vi "Process.vi"(8 "error in":errorcluster, 11 "Framework-Template":refnum<class "Instrument.Framework-Template.lvclass">) -> (0 "error out":errorcluster, 3 "Framework-Template out":refnum<class "Instrument.Framework-Template.lvclass">)   [LabVIEW 2019, in "Instrument.Framework-Template.lvclass"]
doc: "---------------------------------------------------------------\nJKI State Machine Objects™\nhttp://jki.net/state-machine-objects/\nCopyright (C) 2005-2015, JKI <info@jki.net>\nALL RIGHTS RESERVED"
uses:
  Instrument.Framework-Template.lvclass
  <vilib>/JKI/JKI SMO/SMO/SMO.lvclass
  Framework/Instrument/Instrument.lvclass
  C:/Users/patrick/Documents/GitHub/Instrument-Framework/lvsrc/Framework/Instrument Types/SCPI/Instrument.SCPI.lvclass
  C:/Users/patrick/Documents/GitHub/Instrument-Framework/lvsrc/Framework/Instrument/Instrument.lvclass
  C:/Program Files (x86)/National Instruments/LabVIEW 2019/vi.lib/JKI/JKI SMO/SMO/SMO.lvclass
  <userlib>/LevyLab/RemoteControl/RemoteControl/Typedefs/Message--Cluster.ctl
  <userlib>/LevyLab/RemoteControl/RemoteControl/RemoteControl.lvclass
  Typedefs/PrivateEvents--Framework-Template.MessageToProcess.ctl
  Framework/Instrument Types/SCPI/Instrument.SCPI.lvclass
  subsystems/HAL/HAL.lvclass
panel:
  out "Status":string
  out "State History":string
  # "Instrument.Framework-Template"
  # "Framework-Template"
  # "For instructions on how to use the JKI State Machine Objects, examples and video tutorials, visit:\nhttp://jki.net/state-machine-objects/\n\nJKI State Machine Objects™\nhttp://jki.net/state-machine-objects/\nCopyright (C) 2005-2015, JKI <info@jki.net>\nALL RIGHTS RESERVED"
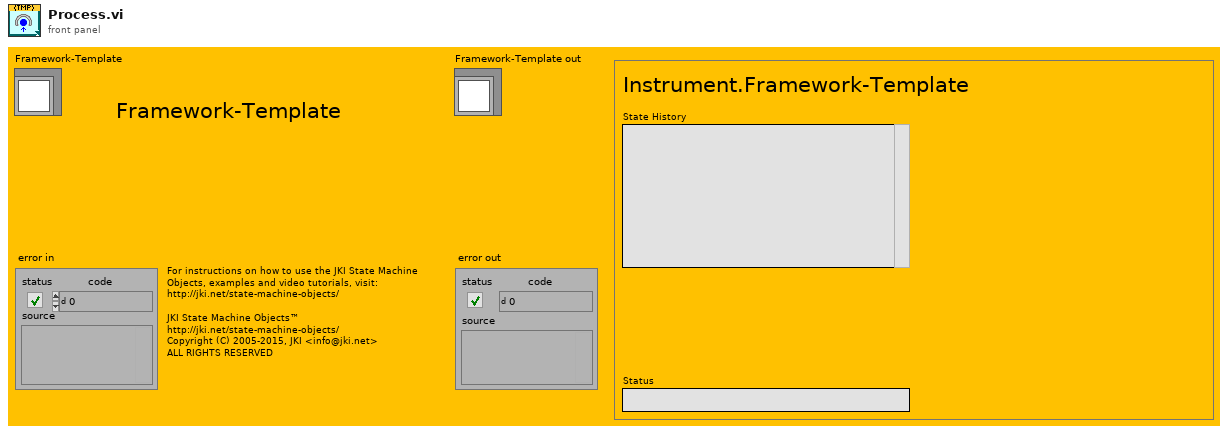
[diagram p1: front panel]
types:
  T1 = enum32{"invalid app kind", "Development System", "Run Time System", "Student Edition", "Embedded LabVIEW", "Evaluation", "Custom"}
  T2 = enum32{"Invalid", "Standard", "Closed", "Hidden", "Minimized", "Maximized"}
  T3 = typedef "RemoteControl.lvclass/Message--Cluster.ctl" = cluster{"Command":string, "Data":variant, "ID":string}
  T4 = typedef "Instrument.Framework-Template.lvclass/PrivateEvents--Framework-Template.MessageToProcess.ctl" = cluster{"Message":T3}
  T5 = cluster{"Core":cluster{"Current VI Reference":refnum<vi>, "Close Panel on Exit?":bool, "Last Error":cluster{"error":errorcluster, "previous state":string, "remaining states":string}, "Shutdown?":bool}, "SelfRef":refnum<class "Instrument.Framework-Template.lvclass">, "HAL":refnum<class "HAL.lvclass">, "Running Step":i32, "sequence":string[], "MessageToProcess":T4}
  T6 = cluster{"Current VI Reference":refnum<vi>, "Close Panel on Exit?":bool, "Last Error":cluster{"error":errorcluster, "previous state":string, "remaining states":string}, "Shutdown?":bool}
  T7 = typedef "SMO.lvclass/Protected Events.ctl" = cluster{"StopProcesses":refnum<user-event>, "AbortProcesses":refnum<user-event>, "Config Changed":refnum<user-event>, "Dependency":refnum<user-event>}
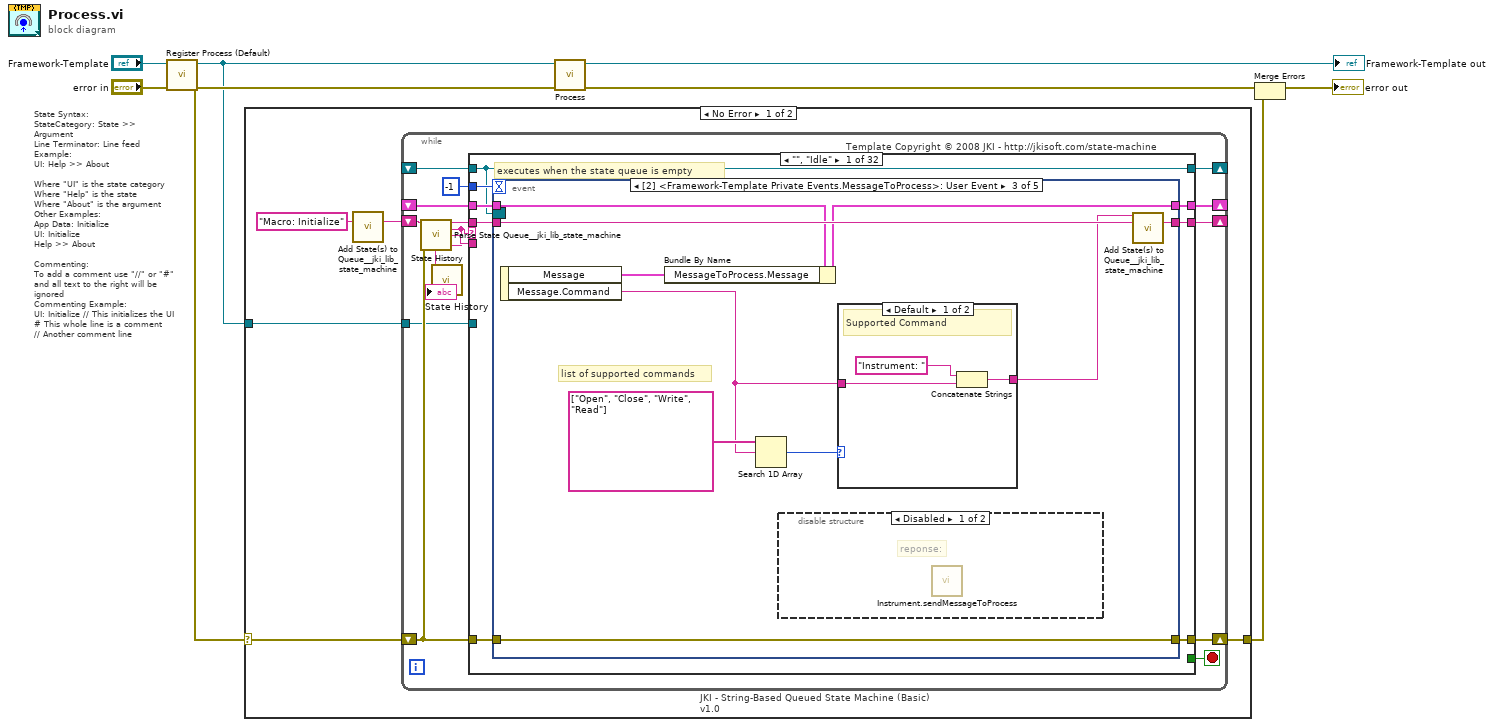
[diagram p0: block diagram]
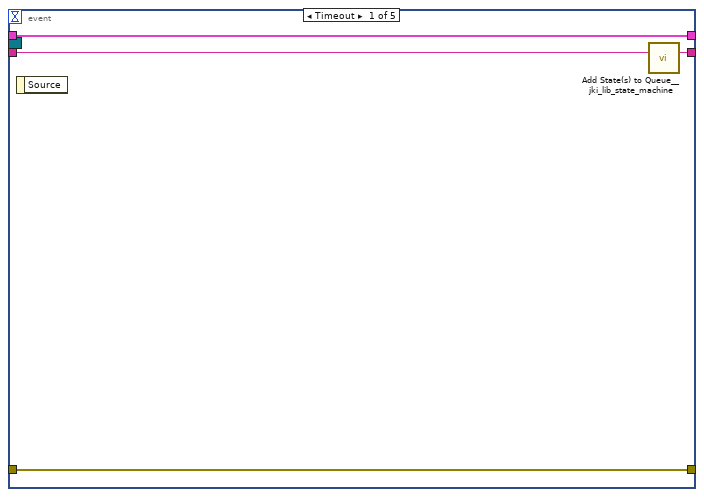
[diagram p2: hidden frame]
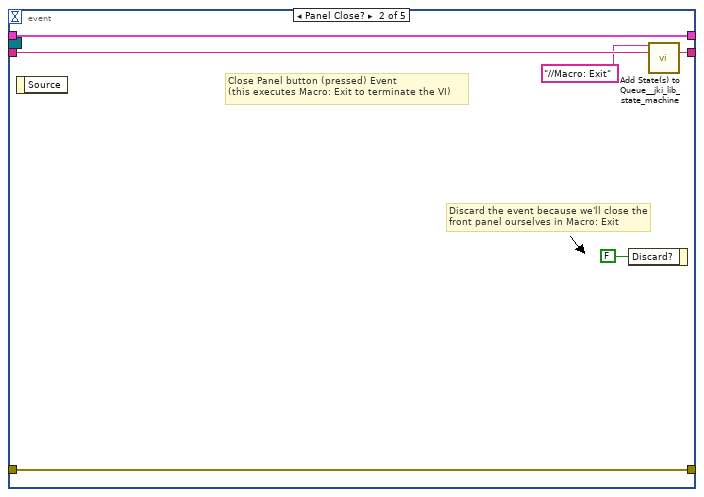
[diagram p3: hidden frame]
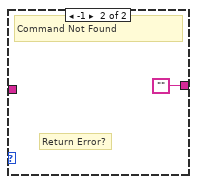
[diagram p5: hidden frame]
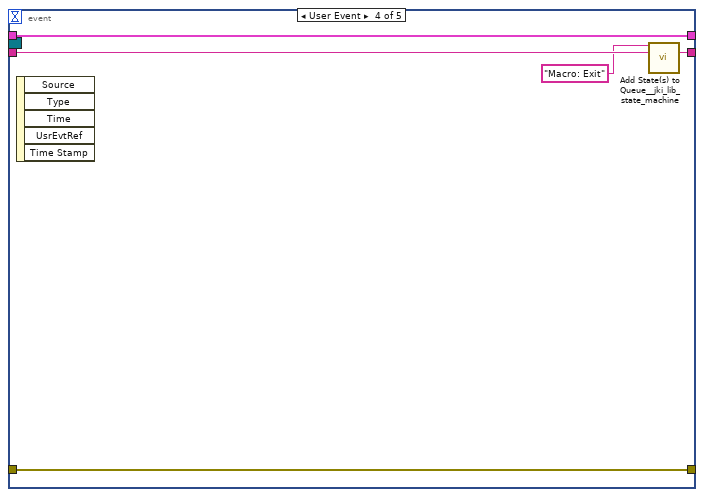
[diagram p6: hidden frame]
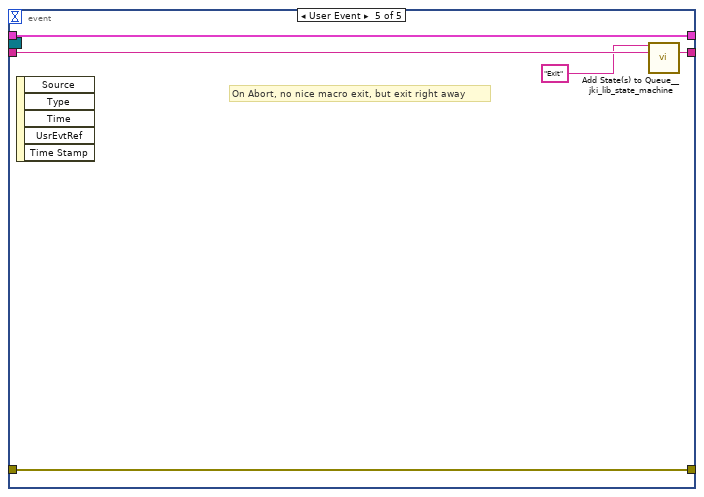
[diagram p7: hidden frame]
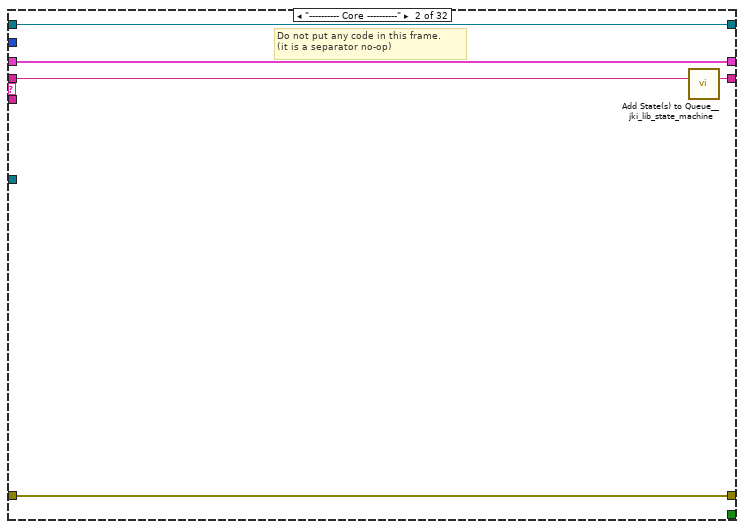
[diagram p8: hidden frame]
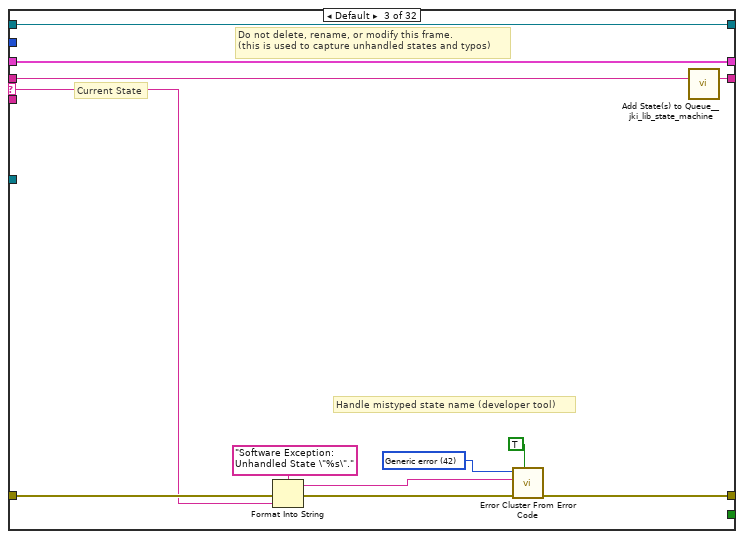
[diagram p9: hidden frame]
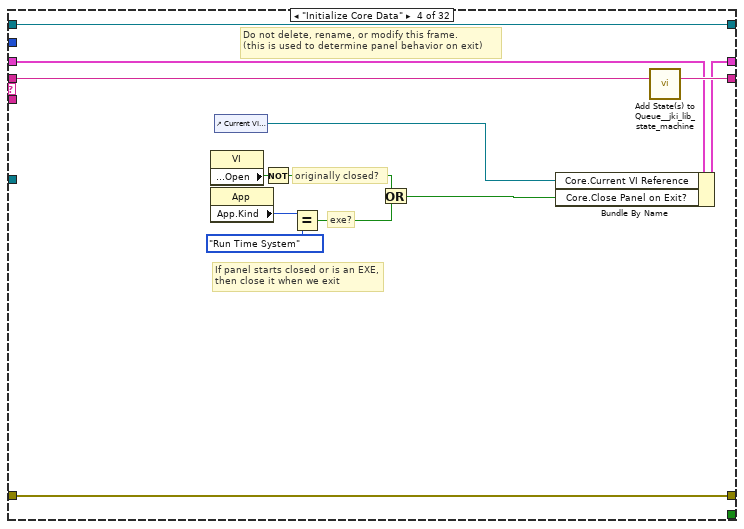
[diagram p10: hidden frame]
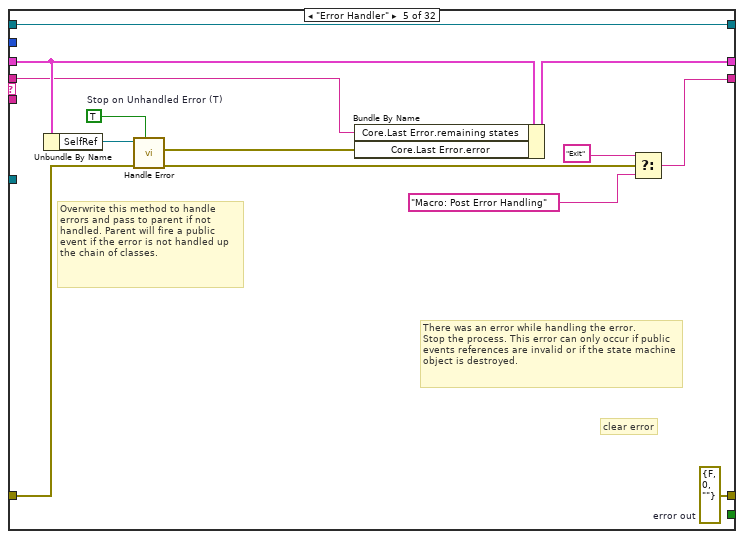
[diagram p11: hidden frame]
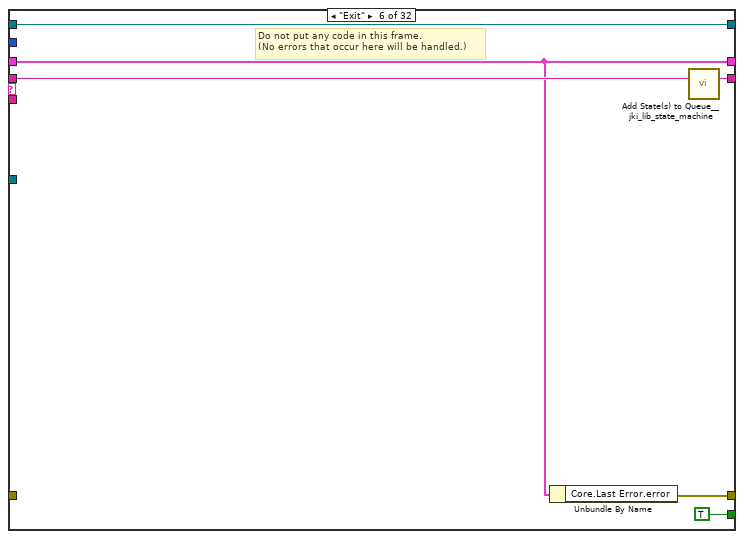
[diagram p12: hidden frame]
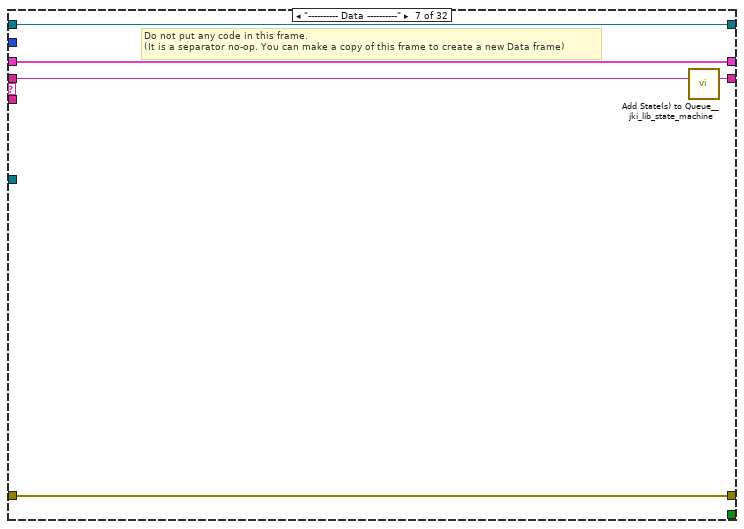
[diagram p13: hidden frame]
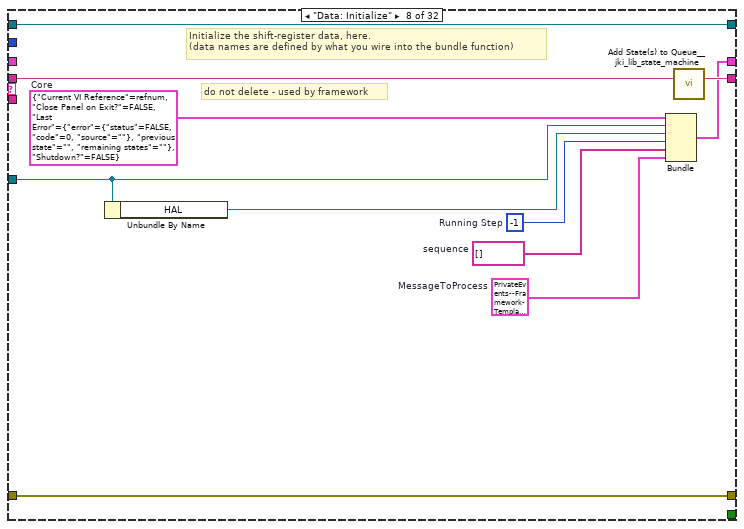
[diagram p14: hidden frame]
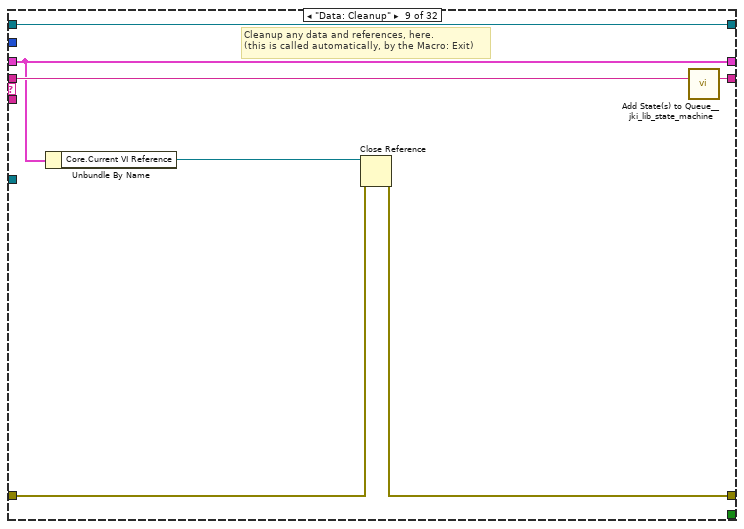
[diagram p15: hidden frame]
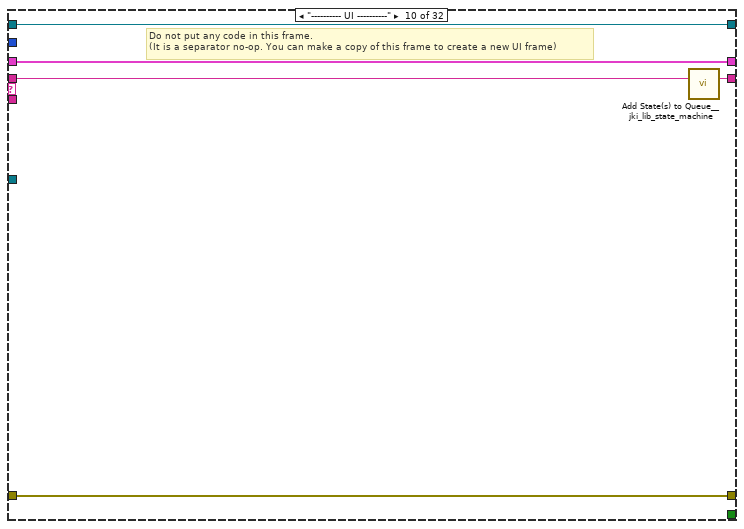
[diagram p16: hidden frame]
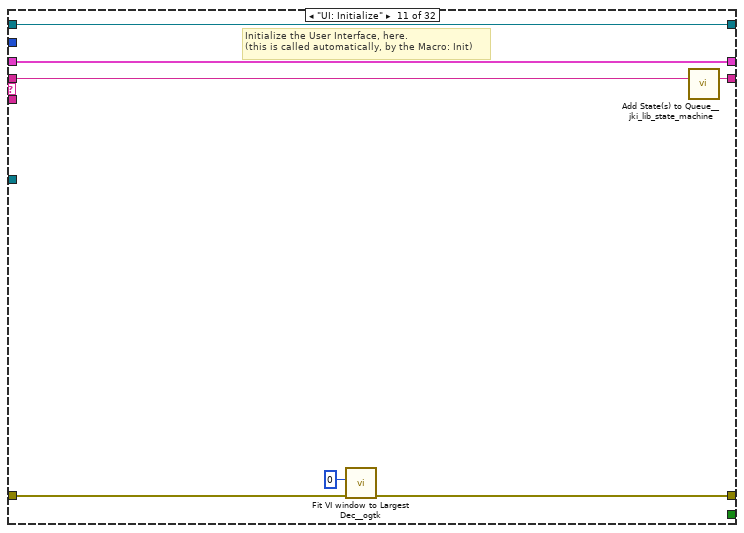
[diagram p17: hidden frame]
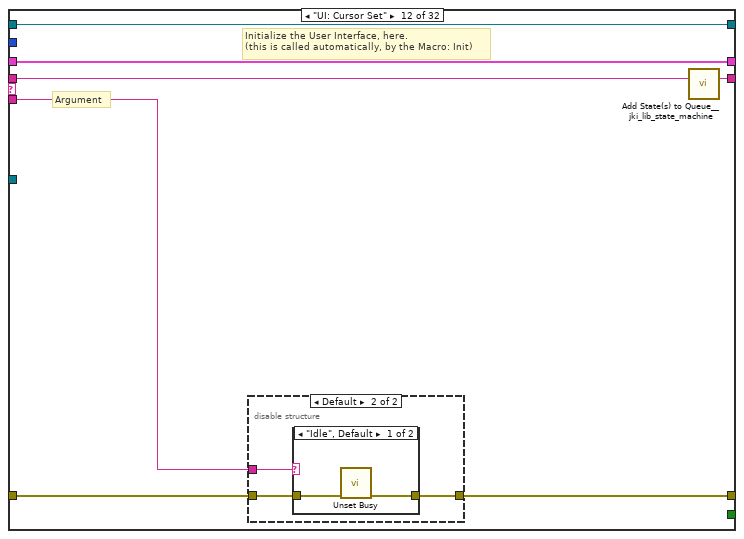
[diagram p18: hidden frame]
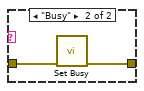
[diagram p20: hidden frame]
diagram:
  # "State Syntax:\nStateCategory: State >> Argument\nLine Terminator: Line feed\nExample:\nUI: Help >> About\n\nWhere \"UI\" is the state category\nWhere \"Help\" is the state\nWhere \"About\" is the argument\nOther Examples:\nApp Data: Initialize\nUI: Initialize\nHelp >> About\n\nCommenting:\nTo add a comment use \"//\" or \"#\" and all text to the right will be ignored\nCommenting Example:\nUI: Initialize // This initializes the UI\n# This whole line is a comment\n// Another comment line"
  n1 = call <vilib>:"Register Process (Default).vi"("error in (no error)"="error in", "SMO"="Framework-Template") -> ("error out"=w5:errorcluster, "SelfRef"=w4:refnum<class "Instrument.Framework-Template.lvclass">)  [unwired: 8 in]
  n2 = case shown="No Error" w5 {
    selector: w5 -> [w10 w422]
    tunnel: w4 -> [w11 _]
    tunnel: [w9 w422] -> w1
    frame No Error {
      n3 = call <vilib>:"Add State(s) to Queue__jki_lib_state_machine.vi"("State(s) in (\"\")"="Macro: Initialize") -> ("States Out"=w13:string)  [unwired: 14 in]
      n4 = while "JKI - String-Based Queued State Machine (Basic) v1.0" {
        shift-right: [w22] -> _
        shift-left: _ -> [w21]
        shift-right: [w25] -> w9
        shift-left: w10 -> [w19]
        shift-right: [w24] -> _
        shift-left: w13 -> [w26]
        tunnel: w11 -> [w18]
        shift-right: [w17] -> _
        shift-left: _ -> [w16]
        stop <- w23 stop-if-true
        # "Template Copyright © 2008 JKI - http://jkisoft.com/state-machine"
        n5 = call <vilib>:"Parse State Queue__jki_lib_state_machine.vi"("State Queue"=w26, "Error In (no error)"=w19) -> ("Remaining States"=w28:string, "Current State"=w15:string, "Arguments"=w27:string)  [unwired: 11 in]
        n6 = call "State History.vi"("Current State"=w15) -> ("History"=→"State History":string)  [unwired: 10 in]
        n7 = case shown="\"\", \"Idle\"" w15 {
          selector: w15 -> [_ _ w77 _ _ _ _ _ _ _ _ _ _ _ _ _ _ _ _ _ _ _ _ _ _ _ _ _ _ _ _ _]
          tunnel: w28 -> [w36 w75 w81 w100 w105 w119 w124 w135 w142 w147 w154 w161 w177 w209 w228 w240 w261 w283 w288 w299 w304 w317 w323 w330 w339 w348 w358 w367 w382 w396 w402 w421]
          tunnel: w27 -> [_ _ _ _ _ _ _ _ _ _ _ w155 w171 _ _ _ _ _ _ _ _ _ _ _ _ _ _ _ _ _ w397 w405]
          tunnel: w21 -> [w34 w72 w79 w91 w109 w115 w121 _ w137 w144 w152 w159 w173 w206 w225 w230 w251 w264 w285 w296 w301 w310 w321 w325 w335 w344 w354 w363 w378 w392 w398 w411]
          tunnel: [w33 w73 w83 w97 w110 w114 w122 w128 w138 w145 w149 w156 w174 w207 w213 w238 w259 w266 w286 w290 w302 w313 w319 w327 w332 w341 w351 w360 w372 w393 w399 w413] -> w25
          tunnel: w19 -> [w32 w73 w82 w97 w111 _ w122 w128 w139 w145 w148 w157 w175 w207 w217 w238 w259 w267 w286 w291 w302 w307 w319 w327 w331 w340 w350 w359 w376 w393 w399 w407]
          tunnel: [w35 w74 w80 w99 w101 w118 w123 w134 w141 w146 w153 w160 w176 w208 w227 w239 w260 w282 w287 w298 w303 w316 w322 w329 w338 w347 w357 w366 w381 w395 w401 w420] -> w24
          tunnel: [_ _ _ _ _ TRUE _ _ _ _ _ _ _ _ _ _ _ _ _ _ _ _ _ _ _ _ _ _ _ _ _ _] -> w23
          tunnel: [w31 w72 w79 w98 w108 w115 w121 w133 w137 w144 w152 w159 w173 w206 w225 w231 w252 w264 w285 w296 w301 w310 w321 w326 w336 w345 w355 w364 w379 w392 w398 w410] -> w22
          tunnel: -1 ("Timeout") -> [w30 _ _ _ _ _ _ _ _ _ _ _ _ _ _ _ _ _ _ _ _ _ _ _ _ _ _ _ _ _ _ _]
          tunnel: w18 -> [_ _ _ _ _ _ _ w126 _ _ _ _ _ _ w221 _ _ w263 _ _ _ _ _ _ _ _ _ _ _ _ _ _]
          tunnel: [w29 w71 w76 w88 w113 w116 w120 w132 w136 w143 w151 w158 w170 w205 w226 w237 w258 w277 w284 w297 w300 w315 w320 w328 w337 w346 w356 w365 w380 w394 w400 w419] -> w17
          tunnel: w16 -> [w29 w71 w76 w88 w113 w116 w120 w132 w136 w143 w151 w158 w170 w205 w226 w237 w258 w277 w284 w297 w300 _ w320 w328 w337 w346 w356 w365 w380 w394 w400 w419]
          frame "", "Idle" {
            # "executes when the state queue is empty"
            n8 = event shown="[2] <Framework-Template Private Events.MessageToProcess>: User Event" {
              selector: w29 -> [_ _ _ _ _]
              dyn-events: _ -> [_ _ _ _ _]
              timeout: w30 -> [_ _ _ _ _]
              tunnel: w36 -> [w40 w46 w56 w65 w70]
              tunnel: [w39 w45 w55 w64 w69] -> w35
              tunnel: w34 -> [w37 w43 w48 w62 w67]
              tunnel: [w38 w44 w54 w63 w68] -> w33
              tunnel: w32 -> [w38 w44 w54 w63 w68]
              tunnel: [w37 w43 w49 w62 w67] -> w31
              event Timeout {
                n9 = event-data() -> ()  [unwired: 1 in, 1 out]
                n10 = call <vilib>:"Add State(s) to Queue__jki_lib_state_machine.vi"("State(s) in (\"\")"=w40) -> ("States Out"=w39:string)  [unwired: 14 in]
              }
              event Panel Close? {
                # "Discard the event because we'll close the front panel ourselves in Macro: Exit"
                # "Close Panel button (pressed) Event\n(this executes Macro: Exit to terminate the VI)"
                n11 = event-data() -> ()  [unwired: 1 in, 1 out]
                n12 = event-data("Discard?"=FALSE) -> ()  [unwired: 1 in, 1 out]
                n13 = call <vilib>:"Add State(s) to Queue__jki_lib_state_machine.vi"("State(s) in Front (\"\")"="//Macro: Exit", "State(s) in (\"\")"=w46) -> ("States Out"=w45:string)  [unwired: 13 in]
              }
              event User Event {
                # "list of supported commands"
                n14 = event-data() -> ("Message"=w47:T3, "Message.Command"=w50:string)  [unwired: 1 in]
                n15 = Bundle By Name(cluster=w48, "MessageToProcess.Message"=w47) -> (w49:T5)
                n16 = Search 1D Array(1D array=string[] ["Open", "Close", "Write", "Read"], element=w50) -> (index of element=w53:i32)  [unwired: 1 in]
                n17 = disable-structure shown="Disabled" {
                  frame Disabled {
                    # "reponse:"
                    n18 = call "Instrument.sendMessageToProcess.vi"() -> ()  [unwired: 10 in, 2 out]
                  }
                  frame Enabled {
                  }
                }
                n19 = case shown="Default" w53 {
                  tunnel: [w59 ""] -> w51
                  tunnel: w50 -> [w58 _]
                  frame Default {
                    # "Supported Command"
                    n20 = Concatenate Strings("Instrument: ", w58) -> (w59:string)
                  }
                  frame -1 {
                    # "Return Error?"
                    # "Command Not Found"
                  }
                }
                n21 = call <vilib>:"Add State(s) to Queue__jki_lib_state_machine.vi"("State(s) in Front (\"\")"=w51, "State(s) in (\"\")"=w56) -> ("States Out"=w55:string)  [unwired: 13 in]
              }
              event User Event {
                n22 = event-data() -> ()  [unwired: 1 in, 5 out]
                n23 = call <vilib>:"Add State(s) to Queue__jki_lib_state_machine.vi"("State(s) in Front (\"\")"="Macro: Exit", "State(s) in (\"\")"=w65) -> ("States Out"=w64:string)  [unwired: 13 in]
              }
              event User Event {
                # "On Abort, no nice macro exit, but exit right away"
                n24 = event-data() -> ()  [unwired: 1 in, 5 out]
                n25 = call <vilib>:"Add State(s) to Queue__jki_lib_state_machine.vi"("State(s) in Front (\"\")"="Exit", "State(s) in (\"\")"=w70) -> ("States Out"=w69:string)  [unwired: 13 in]
              }
            }
          }
          frame "---------- Core ----------" {
            # "Do not put any code in this frame.\n(it is a separator no-op)"
            n26 = call <vilib>:"Add State(s) to Queue__jki_lib_state_machine.vi"("State(s) in (\"\")"=w75) -> ("States Out"=w74:string)  [unwired: 14 in]
          }
          frame Default {
            w86 = 42 items=["No error", "Argument error", "Memory is full", "Out of zone", "End of file", "File already open", "Generic file I/O error", "File not found", "File permission error", "Disk is full", "Duplicate path", "Too many files open", "System feature not enabled", "Resource file not found", "Cannot add resource", "Resource not found", "Image not found", "Image memory error", "Pen does not exist", "Config type invalid", "Config token not found", "Config parse error", "Config memory error", "Bad external code format", "Bad external code offset", "External code not present", "Null window", "Destroy window error", "Null menu", "Print aborted", "Bad print record", "Print driver error", "Windows error during printing", "Memory error during printing", "Print dialog error", "Generic print error", "Invalid device refnum", "Device not found", "Device parameter error", "Device unit error", "Cannot open device", "Device call aborted", "Generic error", "Cancelled by user", "Object ID too low", "Object ID too high", "Object not in heap", "Unknown heap", "Unknown object (invalid DefProc)", "Unknown object (DefProc not in table)", "Message out of range", "Invalid (null) method", "Unknown message", "Manager call not supported", "Bad address", "Network operation in progress", "Network operation timed out", "Connection is busy", "Network attribute not supported", "Network error", "Address in use", "System out of memory", "Connection aborted", "Connection refused", "Not connected", "Already connected", "Connection closed", "Initialization error (interapplication manager)", "Bad occurrence", "Wait on unbound occurrence handler", "Occurrence queue overflow", "Datalog type conflict", "Unused", "Unrecognized type (interapplication manager)", "Memory corrupt", "Failed to make temporary DLL", "Old CIN version", "Drag socket not found", "Failed to load drop-object", "Failed to register OLE object", "Failed to release OLE object", "Format specifier type mismatch", "Unknown format specifier", "Too few format specifiers", "Too many format specifiers", "Scan failed", "Newer CIN version", "Error converting to variant", "Runtime menu error", "Password tampered", "Variant attribute not found", "Incompatible variant data type", "Event data is not available", "Event Store is not present", "Occurrence is not found", "Event Queue is not created", "Event info is not available", "Refnum passed is NULL", "Error retrieving Class GUID", "Error retrieving CoClass GUID", "Error retrieving TypeLib GUID.", "Bad built application magic bytes.", "Specific driver is different from the specific driver associated with the Logical Name.", "There is no session opened to the class driver.", "Max Error", "MAX - Error with config objects", "MAX - Error loading configuration", "MAX - Group not supported"]
            # "Current State"
            # "Do not delete, rename, or modify this frame.\n(this is used to capture unhandled states and typos)"
            # "Handle mistyped state name (developer tool)"
            n27 = Format Into String(format string="Software Exception: Unhandled State \"%s\"." ("message"), error in=w82, w77) -> (resulting string=w85:string, error out=w84:errorcluster)  [unwired: 1 in]
            n28 = call <vilib>:"Error Cluster From Error Code.vi"("show call chain? (False)"=TRUE, "error in (no error)"=w84, "error message (\"\")"=w85, "error code (0)"=w86) -> ("error out"=w83:errorcluster)  [unwired: 5 in]
            n29 = call <vilib>:"Add State(s) to Queue__jki_lib_state_machine.vi"("State(s) in (\"\")"=w81) -> ("States Out"=w80:string)  [unwired: 14 in]
          }
          frame "Initialize Core Data" {
            # "Do not delete, rename, or modify this frame.\n(this is used to determine panel behavior on exit)"
            # "originally closed?"
            # "exe?"
            # "If panel starts closed or is an EXE, then close it when we exit"
            n30 = property class="VI"() -> ("Front Panel.Open"=w96:bool)  [unwired: 2 in, 2 out]
            n31 = property class="App"() -> ("App.Kind"=w95:T1)  [unwired: 2 in, 2 out]
            n32 = control-ref of="Current VI Reference"() -> (w89:refnum<vi>)
            n33 = Not(x=w96) -> (.not. x?=w93:bool)
            n34 = Equal?(x=w95, y=T1."Run Time System" ("Application:Kind")) -> (x = y?=w92:bool)
            n35 = Or(x=w93, y=w92) -> (x .or. y?=w90:bool)
            n36 = Bundle By Name(cluster=w91, "Core.Current VI Reference"=w89, "Core.Close Panel on Exit?"=w90) -> (w98:T5)
            n37 = call <vilib>:"Add State(s) to Queue__jki_lib_state_machine.vi"("State(s) in (\"\")"=w100) -> ("States Out"=w99:string)  [unwired: 14 in]
          }
          frame "Error Handler" {
            w106 = TRUE  # Stop on Unhandled Error (T)
            w110 = errorcluster {"status"=FALSE, "code"=0, "source"=""}  # error out
            # "clear error"
            # "There was an error while handling the error.\nStop the process. This error can only occur if public events references are invalid or if the state machine object is destroyed."
            # "Overwrite this method to handle errors and pass to parent if not handled. Parent will fire a public event if the error is not handled up the chain of classes."
            n38 = Unbundle By Name(w109) -> ("SelfRef"=w112:refnum<class "Instrument.Framework-Template.lvclass">)
            n39 = call-dynamic "Handle Error.vi"("Stop on Unhandled Error (T)"=w106, "error in"=w111, "SMO"=w112) -> ("handling error"=w102:errorcluster, "Unhandled error"=w107:errorcluster)  [unwired: 6 in, 1 out]
            n40 = Bundle By Name(cluster=w109, "Core.Last Error.remaining states"=w105, "Core.Last Error.error"=w107) -> (w108:T5)
            n41 = Select(t="Exit", s=w102, f="Macro: Post Error Handling") -> (s? t:f=w101:string)
          }
          frame "Exit" {
            # "Do not put any code in this frame.\n(No errors that occur here will be handled.)"
            n42 = Unbundle By Name(w115) -> ("Core.Last Error.error"=w114:errorcluster)
            n43 = call <vilib>:"Add State(s) to Queue__jki_lib_state_machine.vi"("State(s) in (\"\")"=w119) -> ("States Out"=w118:string)  [unwired: 14 in]
          }
          frame "---------- Data ----------" {
            # "Do not put any code in this frame.\n(It is a separator no-op. You can make a copy of this frame to create a new Data frame)"
            n44 = call <vilib>:"Add State(s) to Queue__jki_lib_state_machine.vi"("State(s) in (\"\")"=w124) -> ("States Out"=w123:string)  [unwired: 14 in]
          }
          frame "Data: Initialize" {
            w127 = T4 {"Message"={"Command"="", "Data"=variant(string ""), "ID"=""}}  # MessageToProcess
            w129 = string[] []  # sequence
            w130 = -1  # Running Step
            w131 = T6 {"Current VI Reference"=refnum, "Close Panel on Exit?"=FALSE, "Last Error"={"error"={"status"=FALSE, "code"=0, "source"=""}, "previous state"="", "remaining states"=""}, "Shutdown?"=FALSE}  # Core
            # "do not delete - used by framework"
            # "Initialize the shift-register data, here.\n(data names are defined by what you wire into the bundle function)"
            n45 = Unbundle By Name(w126) -> ("HAL"=w125:refnum<class "HAL.lvclass">)
            n46 = Bundle("Core"=w131, "SelfRef"=w126, "HAL"=w125, "Running Step"=w130, "sequence"=w129, "MessageToProcess"=w127) -> (w133:T5)  [unwired: 1 in]
            n47 = call <vilib>:"Add State(s) to Queue__jki_lib_state_machine.vi"("State(s) in (\"\")"=w135) -> ("States Out"=w134:string)  [unwired: 14 in]
          }
          frame "Data: Cleanup" {
            # "Cleanup any data and references, here.\n(this is called automatically, by the Macro: Exit)"
            n48 = Unbundle By Name(w137) -> ("Core.Current VI Reference"=w140:refnum<vi>)
            n49 = Close Reference(reference=w140, error in (no error)=w139) -> (error out=w138:errorcluster)
            n50 = call <vilib>:"Add State(s) to Queue__jki_lib_state_machine.vi"("State(s) in (\"\")"=w142) -> ("States Out"=w141:string)  [unwired: 14 in]
          }
          frame "---------- UI ----------" {
            # "Do not put any code in this frame.\n(It is a separator no-op. You can make a copy of this frame to create a new UI frame)"
            n51 = call <vilib>:"Add State(s) to Queue__jki_lib_state_machine.vi"("State(s) in (\"\")"=w147) -> ("States Out"=w146:string)  [unwired: 14 in]
          }
          frame "UI: Initialize" {
            # "Initialize the User Interface, here.\n(this is called automatically, by the Macro: Init)"
            n52 = call <userlib>:"Fit VI window to Largest Dec__ogtk.vi"("error in (no error)"=w148, "border spacing (2 px)"=0) -> ("error out"=w149:errorcluster)  [unwired: 4 in, 1 out]
            n53 = call <vilib>:"Add State(s) to Queue__jki_lib_state_machine.vi"("State(s) in (\"\")"=w154) -> ("States Out"=w153:string)  [unwired: 14 in]
          }
          frame "UI: Cursor Set" {
            # "Argument"
            # "Initialize the User Interface, here.\n(this is called automatically, by the Macro: Init)"
            n54 = disable-structure shown="Default" {
              disable-tunnel: w157 -> [w162 w165]
              disable-tunnel: [w162 w164] -> w156
              disable-tunnel: w155 -> [_ w163]
              frame condition #0 {
              }
              frame condition #1 (active) {
                n55 = case shown="\"Idle\", Default" w163 {
                  tunnel: w165 -> [w167 w169]
                  tunnel: [w166 w168] -> w164
                  frame "Idle", Default {
                    n56 = call <vilib>:"Unset Busy.vi"("error in (no error)"=w167) -> ("error out"=w166:errorcluster)  [unwired: 10 in]
                  }
                  frame "Busy" {
                    n57 = call <vilib>:"Set Busy.vi"("error in (no error)"=w169) -> ("error out"=w168:errorcluster)  [unwired: 9 in, 1 out]
                  }
                }
              }
            }
            n58 = call <vilib>:"Add State(s) to Queue__jki_lib_state_machine.vi"("State(s) in (\"\")"=w161) -> ("States Out"=w160:string)  [unwired: 14 in]
          }
          frame "UI: Front Panel State" {
            # "Argument"
            # "Set Front Panel Open or Closed\n(Usage: \"UI: Front Panel State >> Open|Close\")"
            n59 = Unbundle By Name(w173) -> ("Core.Current VI Reference"=w172:refnum<vi>)
            n60 = disable-structure shown="TARGET_TYPE==RT" {
              disable-tunnel: w175 -> [w181 w204]
              disable-tunnel: [w180 w204] -> w174
              disable-tunnel: w172 -> [w179 _]
              disable-tunnel: w171 -> [w178 _]
              frame condition #0 (active) {
                n61 = case shown="\"Close\"" w178 {
                  tunnel: w181 -> [w185 w198]
                  tunnel: [w187 w199] -> w180
                  tunnel: w179 -> [w186 w196]
                  frame "Open", Default {
                    n62 = property class="VI"(reference=w186, error in=w185) -> (reference out=w183:refnum<vi>, error out=w184:errorcluster, "FP.State"=w182:T2)
                    n63 = case shown="\"Closed\"" w182 {
                      tunnel: [w190 w193] -> w187
                      tunnel: w184 -> [w189 w193]
                      tunnel: w183 -> [w188 _]
                      frame "Closed" {
                        n64 = invoke class="VI" method="FP.Open"(reference=w188, error in=w189, "Activate"=TRUE, "State"=T2."Standard") -> (error out=w190:errorcluster)  [unwired: 1 in, 4 out]
                      }
                      frame Default {
                      }
                    }
                  }
                  frame "Close" {
                    n65 = property class="VI"(reference=w196, error in=w198) -> (reference out=w195:refnum<vi>, error out=w197:errorcluster, "FP.State"=w194:T2)
                    n66 = case shown="Default" w194 {
                      tunnel: [w200 w203] -> w199
                      tunnel: w197 -> [w200 w202]
                      tunnel: w195 -> [_ w201]
                      frame "Invalid", "Closed" {
                      }
                      frame Default {
                        n67 = invoke class="VI" method="FP.Close"(reference=w201, error in=w202) -> (error out=w203:errorcluster)  [unwired: 1 in, 2 out]
                      }
                    }
                  }
                }
              }
              frame condition #1 {
              }
            }
            n68 = call <vilib>:"Add State(s) to Queue__jki_lib_state_machine.vi"("State(s) in (\"\")"=w177) -> ("States Out"=w176:string)  [unwired: 14 in]
          }
          frame "---------- Macro ----------" {
            # "Do not put any code in this frame.\n(It is a separator no-op. You can make a copy of this frame to create a new Macro frame)"
            n69 = call <vilib>:"Add State(s) to Queue__jki_lib_state_machine.vi"("State(s) in (\"\")"=w209) -> ("States Out"=w208:string)  [unwired: 14 in]
          }
          frame "Macro: Initialize" {
            # "Initialization Macro\n(This is called once, when the VI starts)"
            n70 = call-dynamic "Read Debug Mode.vi"("error in (no error)"=w217, "Instrument in"=w221) -> ("error out"=w216:errorcluster, "Debug Mode?"=w218:bool)  [unwired: 7 in, 1 out]
            n71 = call <userlib>:"Wait (ms)__ogtk.vi"("error in (no error)"=w216, "milliseconds to wait"=u32 0) -> ("error out"=w213:errorcluster)  [unwired: 8 in, 1 out]
            n72 = Select(t="Open", s=w218, f="Close") -> (s? t:f=w214:string)
            n73 = Format Into String(format string="UI: Initialize\nUI: Front Panel State >> %s\nInstrument: Open", initial string="", w214) -> (resulting string=w215:string)  [unwired: 1 in, 1 out]
            n74 = call <vilib>:"Add State(s) to Queue__jki_lib_state_machine.vi"("State(s) in Front (\"\")"="Data: Initialize\nInitialize Core Data\nEvents: Register", "State(s) in (\"\")"="Process: Sync", "State(s) at Back (\"\")"=w215) -> ("States Out"=w223:string)  [unwired: 12 in]
            n75 = call <vilib>:"Add State(s) to Queue__jki_lib_state_machine.vi"("State(s) in Front (\"\")"=w223, "State(s) in (\"\")"=w228) -> ("States Out"=w227:string)  [unwired: 13 in]
          }
          frame "Macro: Post Error Handling" {
            # "Clear Last Error?"
            n76 = Unbundle By Name(w230) -> ("Core.Last Error.remaining states"=w232:string, "Core.Shutdown?"=w233:bool)
            n77 = Unbundle By Name(w230) -> ("Core.Last Error.error"=w236:errorcluster)
            n78 = case shown="False" FALSE {
              tunnel: w236 -> [w244 _]
              tunnel: [w244 _] -> w235
              frame False {
              }
              frame True {
              }
            }
            n79 = case shown="True" w233 {
              tunnel: w232 -> [w241 w243]
              tunnel: [w241 w242] -> w229
              frame False {
                # "These are the remaining states (at the moment the error occured). States can be altered according to business logic."
                # "NOT SHUTTING DOWN"
              }
              frame True {
                # "Developer can decide to alter the states but should be aware that during the shutdown process, there are certain states that must be run for the SMO to properly shut itself (and this process) down. As such, one can add states to perform additional clean-ups, but should append the remaining state to be executed."
                # "SHUTTING DOWN"
                n80 = call <vilib>:"Add State(s) to Queue__jki_lib_state_machine.vi"("State(s) in (\"\")"=w243) -> ("States Out"=w242:string)  [unwired: 14 in]
              }
            }
            n81 = Bundle By Name(cluster=w230, "Core.Last Error.error"=w235) -> (w231:T5)
            n82 = call <vilib>:"Add State(s) to Queue__jki_lib_state_machine.vi"("State(s) in Front (\"\")"=w229, "State(s) in (\"\")"=w240) -> ("States Out"=w239:string)  [unwired: 13 in]
          }
          frame "Macro: Run Sequence" {
            # "0,1,2,3,4,"
            # "5"
            # "Do not put any code in this frame.\n(It is a separator no-op. You can make a copy of this frame to create a new Macro frame)"
            n83 = Unbundle By Name(w251) -> ("sequence"=w247:string[], "Running Step"=w245:i32)
            n84 = Array Size(array=w247) -> (size(s)=w257:i32)
            n85 = Index Array(array=w247, index=w245) -> (element=w246:string)
            n86 = Greater Or Equal?(x=w257, y=w245) -> (x >= y?=w249:bool)
            n87 = Select(t=-1 ("Running Step"), s=w249, f=w245) -> (s? t:f=w256:i32)
            n88 = Bundle By Name(cluster=w251, "Running Step"=w256) -> (w252:T5)
            n89 = Select(t="Sequence: Status >> ...", s=w249, f="Idle //Check Event Structure\nMacro: Run Sequence" ("State(s) at Back (\"\")")) -> (s? t:f=w248:string)
            n90 = call <vilib>:"Add State(s) to Queue__jki_lib_state_machine.vi"("State(s) in Front (\"\")"=w246, "State(s) at Back (\"\")"=w248) -> ("States Out"=w250:string)  [unwired: 13 in]
            n91 = call <vilib>:"Add State(s) to Queue__jki_lib_state_machine.vi"("State(s) in Front (\"\")"=w250, "State(s) in (\"\")"=w261) -> ("States Out"=w260:string)  [unwired: 13 in]
          }
          frame "Macro: Exit" {
            # "Exit Macro\n(This is called once, when the VI exits)"
            n92 = Unbundle By Name(w264) -> ("Core.Close Panel on Exit?"=w281:bool)
            n93 = call-dynamic "Read Debug Mode.vi"("error in (no error)"=w267, "Instrument in"=w263) -> ("error out"=w266:errorcluster, "Debug Mode?"=w265:bool)  [unwired: 7 in, 1 out]
            n94 = Select(t="Open", s=w265, f="Close") -> (s? t:f=w271:string)
            n95 = call <vilib>:"Build State String with Arguments__JKI_lib_State_Machine.vi"("Arguments (\"\")"=w271, "State"="UI: Front Panel State") -> ("State with Arguments"=w268:string)  [unwired: 4 in]
            n96 = Select(t=w268, s=w281, f="") -> (s? t:f=w279:string)
            n97 = call <vilib>:"Add State(s) to Queue__jki_lib_state_machine.vi"("State(s) in Front (\"\")"="Data: Cleanup\nEvents: Unregister", "State(s) in (\"\")"="Process: Sync", "State(s) at Back (\"\")"="Exit") -> ("States Out"=w274:string)  [unwired: 12 in]
            n98 = call <vilib>:"Add State(s) to Queue__jki_lib_state_machine.vi"("State(s) in Front (\"\")"="Instrument: Close", "State(s) in (\"\")"=w279, "State(s) at Back (\"\")"=w274) -> ("States Out"=w278:string)  [unwired: 12 in]
            n99 = call <vilib>:"Add State(s) to Queue__jki_lib_state_machine.vi"("State(s) in Front (\"\")"=w278, "State(s) in (\"\")"=w283) -> ("States Out"=w282:string)  [unwired: 13 in]
          }
          frame "---------- Process ----------" {
            # "Template Separator\n(You can make a copy of, or modify, this frame)"
            n100 = call <vilib>:"Add State(s) to Queue__jki_lib_state_machine.vi"("State(s) in (\"\")"=w288) -> ("States Out"=w287:string)  [unwired: 14 in]
          }
          frame "Process: Sync" {
            n101 = Unbundle By Name(w296) -> ("SelfRef"=w292:refnum<class "Instrument.Framework-Template.lvclass">)
            n102 = call <vilib>:"WaitOnProcessSync.vi"("error in (no error)"=w291, "SMO"=w292) -> ("error out"=w290:errorcluster, "Don't run?"=w295:bool)  [unwired: 7 in, 1 out]
            n103 = Select(t="Data: Cleanup\nEvents: Unregister\nExit", s=w295, f="") -> (s? t:f=w289:string)
            n104 = call <vilib>:"Add State(s) to Queue__jki_lib_state_machine.vi"("State(s) in Front (\"\")"=w289, "State(s) in (\"\")"=w299) -> ("States Out"=w298:string)  [unwired: 13 in]
          }
          frame "---------- Events ----------" {
            # "Template Separator\n(You can make a copy of, or modify, this frame)"
            n105 = call <vilib>:"Add State(s) to Queue__jki_lib_state_machine.vi"("State(s) in (\"\")"=w304) -> ("States Out"=w303:string)  [unwired: 14 in]
          }
          frame "Events: Register" {
            n106 = Unbundle By Name(w310) -> ("SelfRef"=w311:refnum<class "Instrument.Framework-Template.lvclass">)
            n107 = call <vilib>:"GetProtectedEvents.vi"("SMO"=w311) -> ("error out"=w309:errorcluster, "SMO Protected Events"=w314:T7, "SMO out"=w308:refnum<class "Instrument.Framework-Template.lvclass">)  [unwired: 8 in]
            n108 = call "Instrument-Template.GetPrivateEvents.vi"("Instrument.Framework-Template in"=w308) -> ("error out"=w305:errorcluster, "Framework-Template Private Events"=w306:cluster{"MessageToProcess":refnum<user-event>})  [unwired: 8 in, 1 out]
            n109 = register-events(w314, w306) -> (reference out=w315:refnum<event-registration>, error out=w312:errorcluster)  [unwired: 2 in]
            n110 = Merge Errors(w312, w305, w309, w307) -> (w313:errorcluster)
            n111 = call <vilib>:"Add State(s) to Queue__jki_lib_state_machine.vi"("State(s) in (\"\")"=w317) -> ("States Out"=w316:string)  [unwired: 14 in]
          }
          frame "Events: Unregister" {
            n112 = Unregister For Events(event registration refnum=w320, error in=w319) -> (error out=w318:errorcluster)
            n113 = call <vilib>:"Clear Errors.vi"("error in (no error)"=w318) -> ()  [unwired: 5 in, 2 out]
            n114 = call <vilib>:"Add State(s) to Queue__jki_lib_state_machine.vi"("State(s) in (\"\")"=w323) -> ("States Out"=w322:string)  [unwired: 14 in]
          }
          frame "---------- Instrument ----------" {
            n115 = Unbundle By Name(w325) -> ("HAL"=w324:refnum<class "HAL.lvclass">)
            n116 = Bundle By Name(cluster=w325, "HAL"=w324) -> (w326:T5)
            n117 = call <vilib>:"Add State(s) to Queue__jki_lib_state_machine.vi"("State(s) in (\"\")"=w330) -> ("States Out"=w329:string)  [unwired: 14 in]
          }
          frame "Instrument: Open" {
            n118 = Unbundle By Name(w335) -> ("HAL"=w334:refnum<class "HAL.lvclass">)
            n119 = call-dynamic "Open.vi"("error in (no error)"=w331, "HAL in"=w334) -> ("error out"=w332:errorcluster, "HAL out"=w333:refnum<class "HAL.lvclass">)  [unwired: 8 in]
            n120 = Bundle By Name(cluster=w335, "HAL"=w333) -> (w336:T5)
            n121 = call <vilib>:"Add State(s) to Queue__jki_lib_state_machine.vi"("State(s) in (\"\")"=w339) -> ("States Out"=w338:string)  [unwired: 14 in]
          }
          frame "Instrument: Write" {
            n122 = Unbundle By Name(w344) -> ("HAL"=w343:refnum<class "HAL.lvclass">)
            n123 = call-dynamic "Write.vi"("error in (no error)"=w340, "HAL in"=w343) -> ("error out"=w341:errorcluster, "HAL out"=w342:refnum<class "HAL.lvclass">)  [unwired: 8 in]
            n124 = Bundle By Name(cluster=w344, "HAL"=w342) -> (w345:T5)
            n125 = call <vilib>:"Add State(s) to Queue__jki_lib_state_machine.vi"("State(s) in (\"\")"=w348) -> ("States Out"=w347:string)  [unwired: 14 in]
          }
          frame "Instrument: Read" {
            n126 = Unbundle By Name(w354) -> ("HAL"=w353:refnum<class "HAL.lvclass">)
            n127 = call-dynamic "Read.vi"("error in (no error)"=w350, "HAL in"=w353) -> ("error out"=w351:errorcluster, "response"=w349:string, "HAL out"=w352:refnum<class "HAL.lvclass">)  [unwired: 7 in]
            n128 = Bundle By Name(cluster=w354, "HAL"=w352, "MessageToProcess.Message.Data"=w349) -> (w355:T5)
            n129 = call <vilib>:"Add State(s) to Queue__jki_lib_state_machine.vi"("State(s) in (\"\")"=w358) -> ("States Out"=w357:string)  [unwired: 14 in]
          }
          frame "Instrument: Close" {
            n130 = Unbundle By Name(w363) -> ("HAL"=w362:refnum<class "HAL.lvclass">)
            n131 = call-dynamic "Close.vi"("error in (no error)"=w359, "HAL in"=w362) -> ("error out"=w360:errorcluster, "HAL out"=w361:refnum<class "HAL.lvclass">)  [unwired: 8 in]
            n132 = Bundle By Name(cluster=w363, "HAL"=w361) -> (w364:T5)
            n133 = call <vilib>:"Add State(s) to Queue__jki_lib_state_machine.vi"("State(s) in (\"\")"=w367) -> ("States Out"=w366:string)  [unwired: 14 in]
          }
          frame "Instrument: Do Something" {
            # "communicate with\nhardware"
            n134 = Unbundle By Name(w378) -> ("SelfRef"=w377:refnum<class "Instrument.Framework-Template.lvclass">, "MessageToProcess.Message.Data"=w375:variant, "MessageToProcess.Message.ID"=w370:string)
            n135 = call "Instrument-Template.doSomethingExample.vi"("error in (no error)"=w376, "Data"=w375, "Instrument.Framework-Template in"=w377) -> ("error out"=w371:errorcluster, "Data out"=w369:variant, "Instrument.Framework-Template out"=w374:refnum<class "Instrument.Framework-Template.lvclass">)  [unwired: 6 in]
            n136 = Empty String/Path?(string/path=w369) -> (empty?=w368:bool)
            n137 = case shown="False" w368 {
              tunnel: w374 -> [w389 w391]
              tunnel: [w388 w391] -> w373
              tunnel: [w387 w390] -> w372
              tunnel: w369 -> [w384 _]
              tunnel: w371 -> [w383 w390]
              tunnel: w370 -> [w385 _]
              frame False {
                # "send data to\ninstrument:process.vi"
                n138 = call "Instrument.sendMessageToProcess.vi"("ID"=w385, "error in (no error)"=w383, "Data"=w384, "Command"="Set Parameter", "Instrument"=w389) -> ("error out"=w387:errorcluster, "Instrument out"=w388:refnum<class "Instrument.Framework-Template.lvclass">)  [unwired: 5 in]
              }
              frame True {
              }
            }
            n139 = Bundle By Name(cluster=w378, "SelfRef"=w373) -> (w379:T5)
            n140 = call <vilib>:"Add State(s) to Queue__jki_lib_state_machine.vi"("State(s) in (\"\")"=w382) -> ("States Out"=w381:string)  [unwired: 14 in]
          }
          frame "---------- Sequence ----------" {
            n141 = call <vilib>:"Add State(s) to Queue__jki_lib_state_machine.vi"("State(s) in (\"\")"=w396) -> ("States Out"=w395:string)  [unwired: 14 in]
          }
          frame "Sequence: Status" {
            # "Sequence: Status\n(Use this frame to pass the status to the UI, this VI's UI, etc)"
            n142 = call <vilib>:"Add State(s) to Queue__jki_lib_state_machine.vi"("State(s) in (\"\")"=w402) -> ("States Out"=w401:string)  [unwired: 14 in]
            "Status" <- w397
          }
          frame "Sequence: Wait" {
            # "Sequence: Wait\n(Non-Blocking Wait)"
            # "F = repeat this state. wait\nT = go to next state. don't wait"
            n143 = Unbundle By Name(w411) -> ("Running Step"=w404:i32)
            n144 = call "Wait Logic.vi"("error in (no error)"=w407, "Time"=w405) -> ("error out"=w406:errorcluster, "Status String"=w403:string, "Trigger"=w408:bool)  [unwired: 6 in, 1 out]
            n145 = Increment(x=w404) -> (x+1=w418:i32)
            n146 = Select(t=w418, s=w408, f=w404) -> (s? t:f=w409:i32)
            n147 = Select(t=u32 0, s=w408, f=u32 100 ("milliseconds to wait")) -> (s? t:f=w415:u32)
            n148 = call <userlib>:"Wait (ms)__ogtk.vi"("error in (no error)"=w406, "milliseconds to wait"=w415) -> ("error out"=w413:errorcluster)  [unwired: 8 in, 1 out]
            n149 = Bundle By Name(cluster=w411, "Running Step"=w409) -> (w410:T5)
            n150 = call <vilib>:"Build State String with Arguments__JKI_lib_State_Machine.vi"("Arguments (\"\")"=w403, "State"="Sequence: Status") -> ("State with Arguments"=w412:string)  [unwired: 4 in]
            n151 = call <vilib>:"Add State(s) to Queue__jki_lib_state_machine.vi"("State(s) in Front (\"\")"=w412, "State(s) in (\"\")"=w421) -> ("States Out"=w420:string)  [unwired: 13 in]
          }
        }
      }
    }
    frame Error {
    }
  }
  n152 = call-parent "Process.vi"("error in"=w5, "Instrument"=w4) -> ("error out"=w2:errorcluster, "Instrument out"=→"Framework-Template out":refnum<class "Instrument.Framework-Template.lvclass">)  [unwired: 8 in]
  n153 = Merge Errors(w2, w1) -> (→"error out":errorcluster)
